vi "insert-scecmd-list.vi"(10 "场景":T2, 11 "场景-cmd-list":T1(array[cluster])) -> (3 "场景-cmd-list out":T1(array[cluster]))   [LabVIEW 2019]
panel:
  out "场景 2":T2
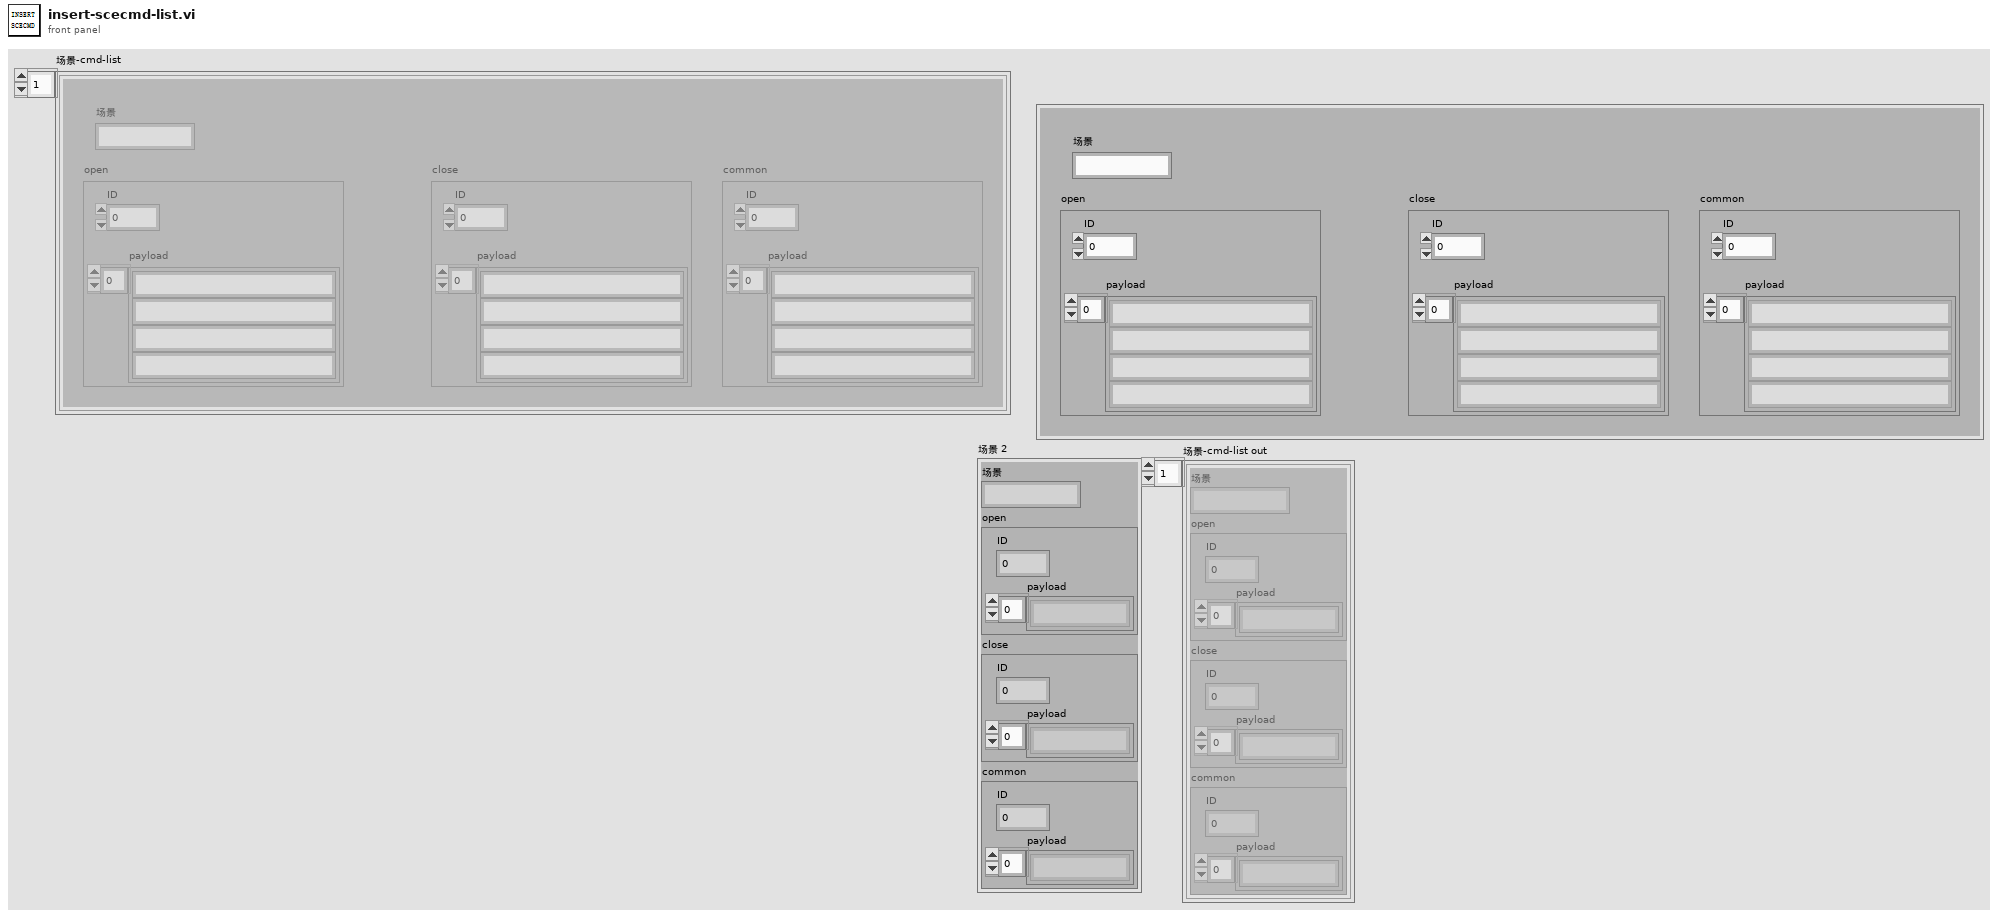
[diagram p1: front panel]
types:
  T1 = cluster{"场景":string, "open":cluster{"ID":dbl, "payload":string[]}, "close":cluster{"ID":dbl, "payload":string[]}, "common":cluster{"ID":dbl, "payload":string[]}}[]
  T2 = cluster{"场景":string, "open":cluster{"ID":dbl, "payload":string[]}, "close":cluster{"ID":dbl, "payload":string[]}, "common":cluster{"ID":dbl, "payload":string[]}}
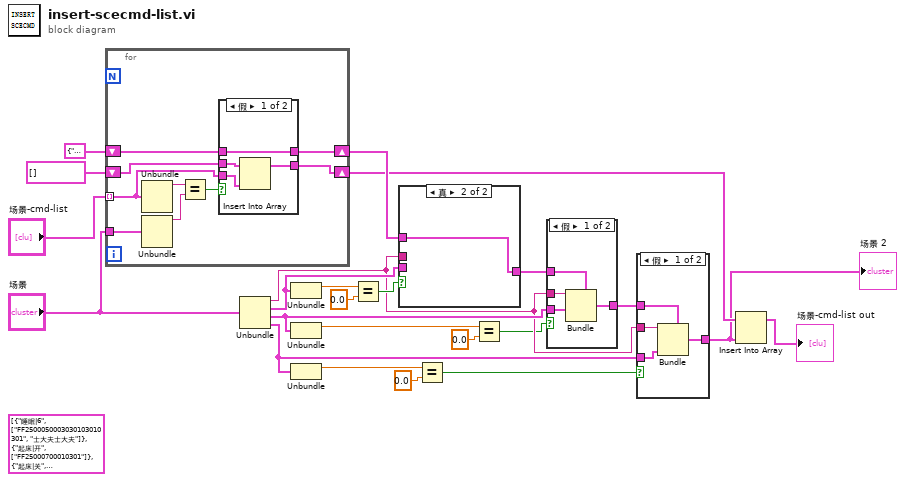
[diagram p0: block diagram]
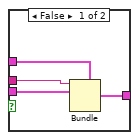
[diagram p4: hidden frame]
diagram:
  (unwired) cluster{"字符串":string, "数组 2":string[]}[] [{"字符串"="睡眠|6", "数组 2"=["FF2500050003030103010301", "士大夫士大夫"]}, {"字符串"="起床|开", "数组 2"=["FF25000700010301"]}, {"字符串"="起床|关", "数组 2"=["FF250006000203010100"]}] ("sce-cmd-list")
  n1 = for {
    tunnel: "场景-cmd-list" -> [w28] mode=indexing
    tunnel: "场景" -> [w32]
    shift-right: [w27] -> w3
    shift-left: T1 [] -> [w26]
    shift-right: [w25] -> w12
    shift-left: T2 {"场景"="", "open"={"ID"=0.0, "payload"=[]}, "close"={"ID"=0.0, "payload"=[]}, "common"={"ID"=0.0, "payload"=[]}} ("场景") -> [w24]
    n2 = Unbundle(w28) -> ("场景"=w31:string)  [unwired: 3 out]
    n3 = Unbundle(w32) -> ("场景"=w30:string)  [unwired: 3 out]
    n4 = Equal?(x=w31, y=w30) -> (x = y?=w29:bool)
    n5 = case shown="假" w29 {
      tunnel: w28 -> [w36 w37]
      tunnel: [w35 w38] -> w27
      tunnel: w26 -> [w34 w38]
      tunnel: [w33 w37] -> w25
      tunnel: w24 -> [w33 _]
      frame False {
        n6 = Insert Into Array(array=w34, new element=w36) -> (w35:T1)  [unwired: 1 in]
      }
      frame True {
      }
    }
  }
  n7 = Unbundle("场景") -> ("场景"=w7:string, "open"=w11:cluster{"ID":dbl, "payload":string[]}, "close"=w9:cluster{"ID":dbl, "payload":string[]}, "common"=w6:cluster{"ID":dbl, "payload":string[]})
  n8 = Unbundle(w11) -> ("ID"=w19:dbl)  [unwired: 1 out]
  n9 = Unbundle(w9) -> ("ID"=w16:dbl)  [unwired: 1 out]
  n10 = Unbundle(w6) -> ("ID"=w15:dbl)  [unwired: 1 out]
  n11 = Equal?(x=w19, y=0.0) -> (x = y?=w13:bool)
  n12 = case shown="真" w13 {
    tunnel: w12 -> [w42 w43]
    tunnel: w7 -> [w41 _]
    tunnel: w11 -> [w40 _]
    tunnel: [w39 w43] -> w10
    frame False {
      n13 = Bundle(cluster=w42, "场景"=w41, "open"=w40) -> (w39:T2)  [unwired: 2 in]
    }
    frame True {
    }
  }
  n14 = Equal?(x=w15, y=0.0) -> (x = y?=w4:bool)
  n15 = Equal?(x=w16, y=0.0) -> (x = y?=w5:bool)
  n16 = case shown="假" w5 {
    tunnel: w10 -> [w47 w48]
    tunnel: w7 -> [w46 _]
    tunnel: w9 -> [w44 _]
    tunnel: [w45 w48] -> w8
    frame False {
      n17 = Bundle(cluster=w47, "场景"=w46, "close"=w44) -> (w45:T2)  [unwired: 2 in]
    }
    frame True {
    }
  }
  n18 = case shown="假" w4 {
    tunnel: w8 -> [w52 w53]
    tunnel: w7 -> [w51 _]
    tunnel: w6 -> [w49 _]
    tunnel: [w50 w53] -> w2
    frame False {
      n19 = Bundle(cluster=w52, "场景"=w51, "common"=w49) -> (w50:T2)  [unwired: 2 in]
    }
    frame True {
    }
  }
  "场景 2" <- w2
  n20 = Insert Into Array(array=w3, new element=w2) -> (→"场景-cmd-list out":T1)  [unwired: 1 in]
